vi "MtrPowerAnalog.vi"(9 "MtrPWR":dbl(knob) scale=-1.0..1.0, 11 "PwrON":bool) -> (3 "MtrPWR":dbl)   [LabVIEW 2015]
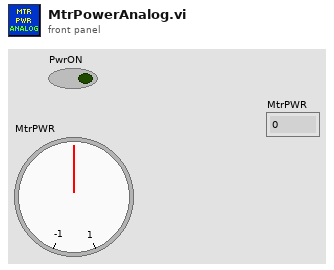
[diagram p1: front panel]
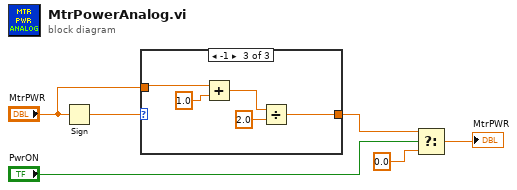
[diagram p0: block diagram]
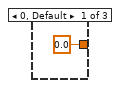
[diagram p2: hidden frame]
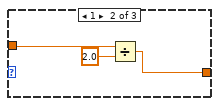
[diagram p3: hidden frame]
diagram:
  n1 = Sign(1:"MtrPWR") -> (0:w4:dbl)
  n2 = case shown="-1" w4 {
    tunnel: "MtrPWR" -> [_ w10 w15]
    tunnel: [0.0 w9 w11] -> w2
    frame 0, Default {
    }
    frame 1 {
      n3 = Divide(x=w10, y=2.0) -> (x/y=w9:dbl)
    }
    frame -1 {
      n4 = Add(x=w15, y=1.0) -> (x+y=w13:dbl)
      n5 = Divide(x=w13, y=2.0) -> (x/y=w11:dbl)
    }
  }
  n6 = Select(t=w2, s="PwrON", f=0.0) -> (s? t:f=→"MtrPWR":dbl)
